vi "Initialize.vi"(8 "error in (no error)":errorcluster, 11 "IMAQdx Camera in":refnum<class "IMAQdx Camera.lvclass">) -> (0 "error out":errorcluster, 3 "IMAQdx Camera out":refnum<class "IMAQdx Camera.lvclass">)   [LabVIEW 2011, in "IMAQdx Camera.lvclass"]
uses:
  IMAQdx Camera.lvclass
  Camera Class/Camera.lvclass
  <vilib>/vision/driver/IMAQdx.llb/IMAQdx Camera Control Mode.ctl
  IMAQdx Camera.lvclass/IMAQdx Camera.ctl
  <vilib>/vision/driver/NI_Vision_Acquisition_Software.lvlib
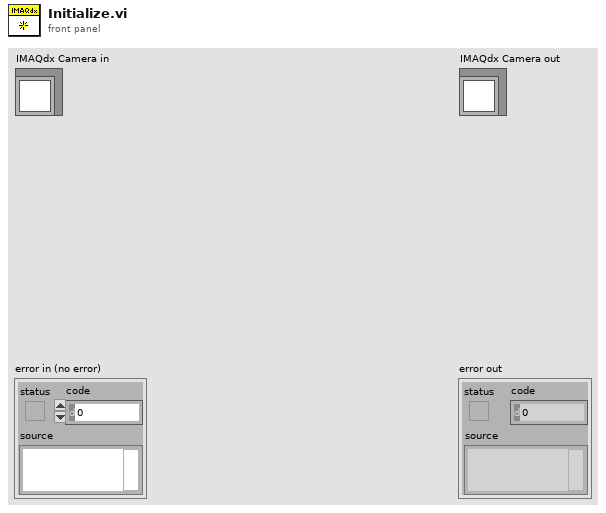
[diagram p1: front panel]
types:
  T1 = typedef "NI_Vision_Acquisition_Software.lvlib/IMAQdx Camera Control Mode.ctl" = enum32{"Controller", "Listener"}
  T2 = typedef "IMAQdx.ctl" = refnum<k21>
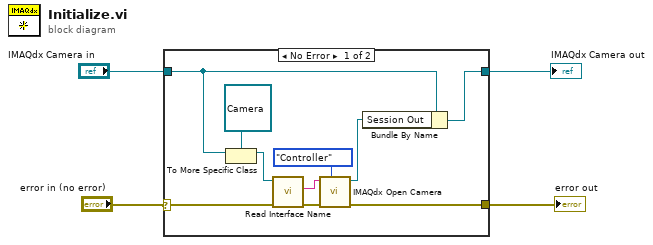
[diagram p0: block diagram]
diagram:
  n1 = case shown="No Error" "error in (no error)" {
    selector: "error in (no error)" -> [w5 w16]
    tunnel: "IMAQdx Camera in" -> [w8 w15]
    tunnel: [w7 w15] -> w3
    tunnel: [w6 w16] -> w2
    frame No Error {
      n2 = To More Specific Class(target class=refnum<class "Camera.lvclass"> refnum ("Image UDP Broadcast Custom Device.lvlib:Camera.lvclass"), reference=w8) -> (specific class reference=w12:refnum<class "Camera.lvclass">)  [unwired: 1 in, 1 out]
      n3 = call-dynamic "Read Interface Name.vi"("error in (no error)"=w5, "Camera in"=w12) -> ("error out"=w10:errorcluster, "Interface Name"=w11:string)  [unwired: 7 in, 1 out]
      n4 = call <vilib>:"IMAQdx Open Camera.vi"("Camera Control Mode"=IMAQdx_Camera_Control_Mode."Controller", "error in"=w10, "Session In"=w11) -> ("error out"=w6:errorcluster, "Session Out"=w9:T2)  [unwired: 7 in]
      n5 = Bundle By Name(cluster=w8, "Session Out"=w9) -> (w7:refnum<class "IMAQdx Camera.lvclass">)
    }
    frame Error {
    }
  }
  "error out" <- w2
  "IMAQdx Camera out" <- w3
